vi "Save_Time_Traces_HACKforPWLDA.vi"() -> (5 "Plug in titles":string[](array[string]), 7 "Plug in values":string[](array[string]))   [LabVIEW 2010]
uses:
  Plug in sub vis/save_time _trace.ctl
  Globals/Meas_global.vi
  Globals/Plug_in_data_global.vi
  Acquisition/PWA/PWAtasksGLOBAL.vi
  Globals/LDA_meas_global_1.vi
panel:
  in  "Time Series":enum16{"Milliseconds", "Seconds"}(ring)
  in  "Full Header Info?":bool
  in  "Data Type":T1
  in  "Output Directory":path
  in  "Put each block into separate file":bool
  in  "Leave space between blocks?":bool
  in  "Precision":i16=2
  in  "Data to save":i32[](array[ring])=[1] items=["Preston (1)", "Save Nothing"]
  in  "Separation Character":string="\t"
  # "Run this VI to update the channel names"
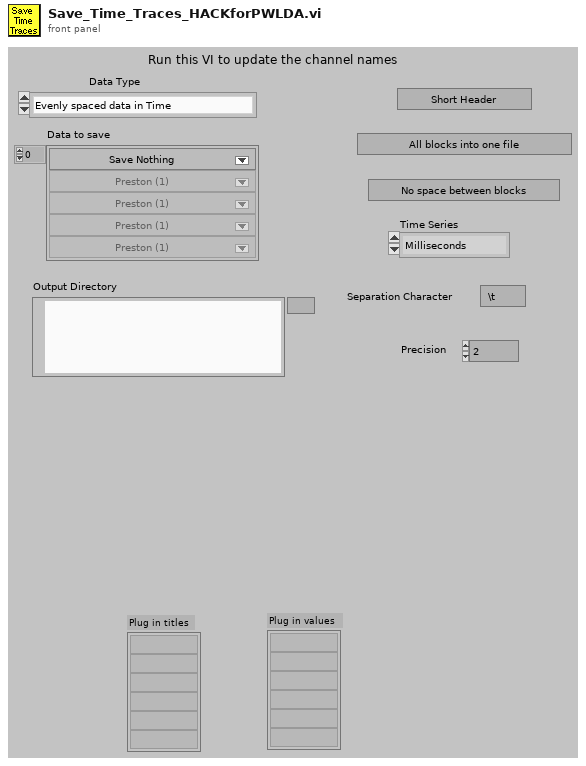
[diagram p1: front panel]
types:
  T1 = typedef "save_time _trace.ctl" = enum16{"Evenly spaced data in Time", "Unevenly spaced data in Time", "Pulsed Wire data"}
  T2 = typedef "Analysis_info_cluster.ctl" = cluster{"Colour":u32, "Inst type":T3, "Inst name":string, "Symbol":string, "Code name":string, "Extra Info":string, "Inst Array":T4, "Index":i32, "Voltage Index":i32, "Extra Titles":string[], "Extra Values":string[]}
  T3 = typedef "Inst_type.ctl" = enum16{"Propeller anemometer", "Raw voltage", "Pressure Transducer", "Pitot-static tube", "Preston tube", "Hot wire", "Cross wire 1", "Cross wire 2", "Generic Linear", "Generic Polynomial", "Generic BackPoly", "Fast FID", "Thermocouple", "Cold wire", "Pulsed Wire", "LDA Vel", "LDA Tran time", "LDA Arr time"}
  T4 = typedef "Instrument_Array.ctl" = enum16{"PWA", "LDA", "Analogue"}
  T5 = enum32{"existing file", "new file", "new or existing file", "existing dir", "new dir", "new or existing dir", "existing file (use LLBs)", "new file (use LLBs)", "new or existing file (use LLBs)", "new or existing file or directory (use LLBs)"}
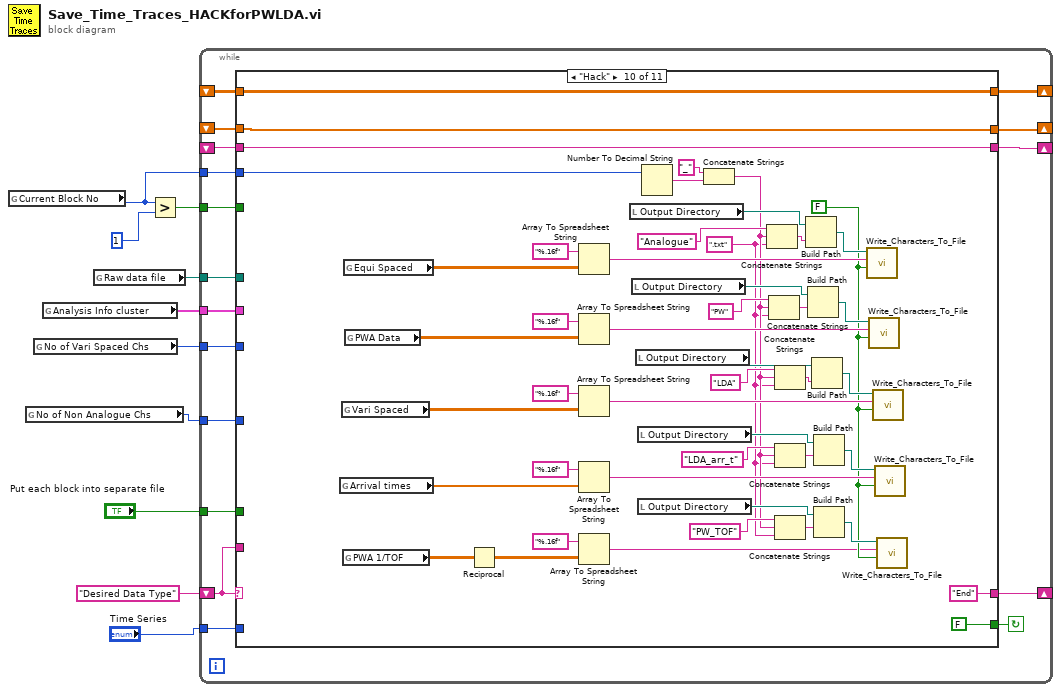
[diagram p0: block diagram]
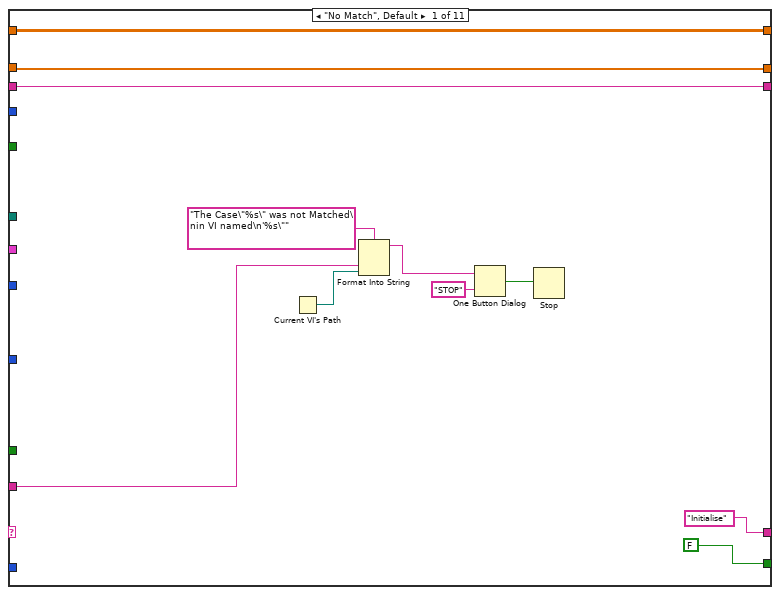
[diagram p2: hidden frame]
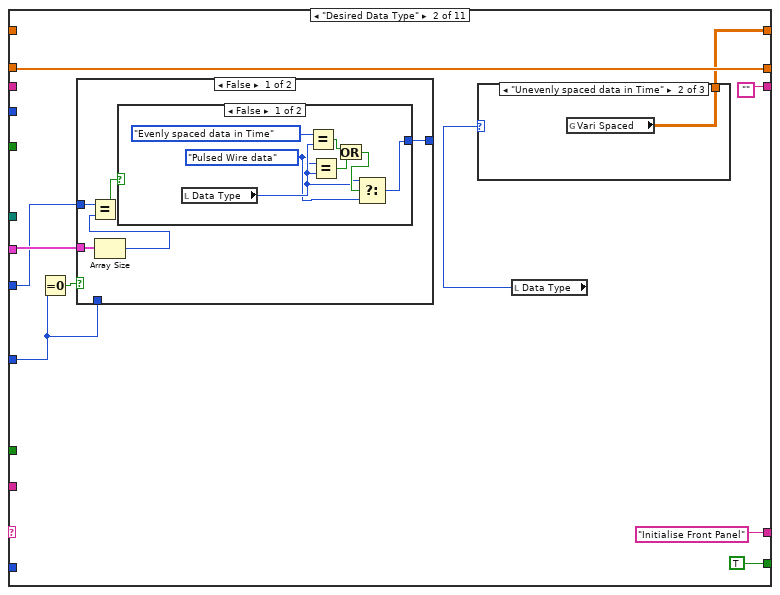
[diagram p3: hidden frame]
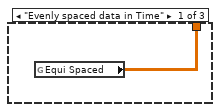
[diagram p4: hidden frame]
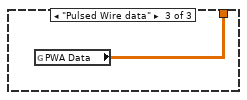
[diagram p5: hidden frame]
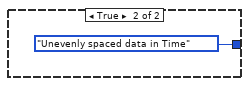
[diagram p6: hidden frame]
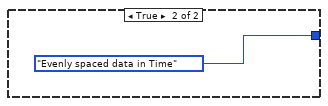
[diagram p7: hidden frame]
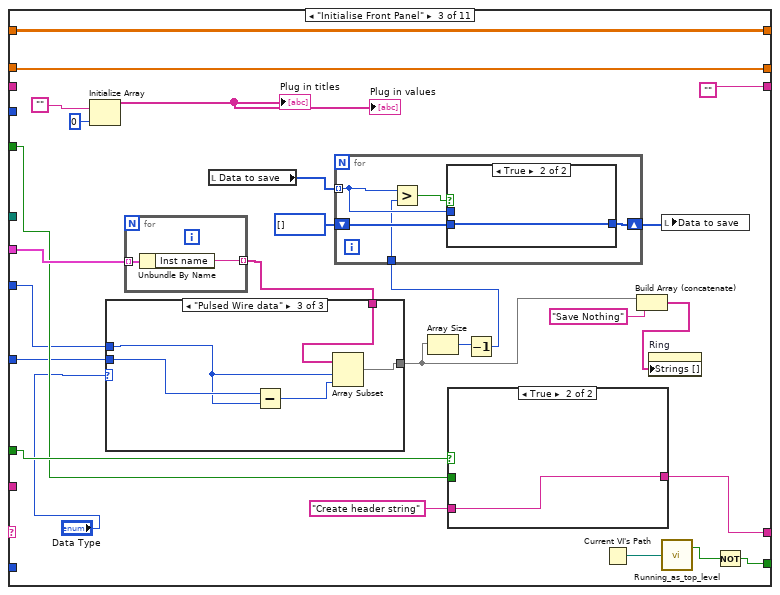
[diagram p8: hidden frame]
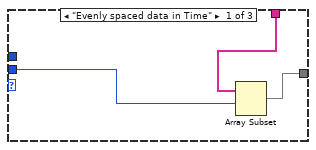
[diagram p9: hidden frame]
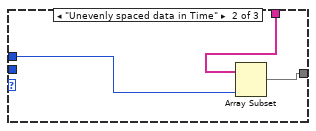
[diagram p10: hidden frame]
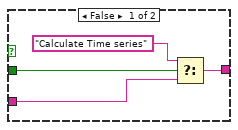
[diagram p11: hidden frame]
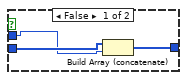
[diagram p12: hidden frame]
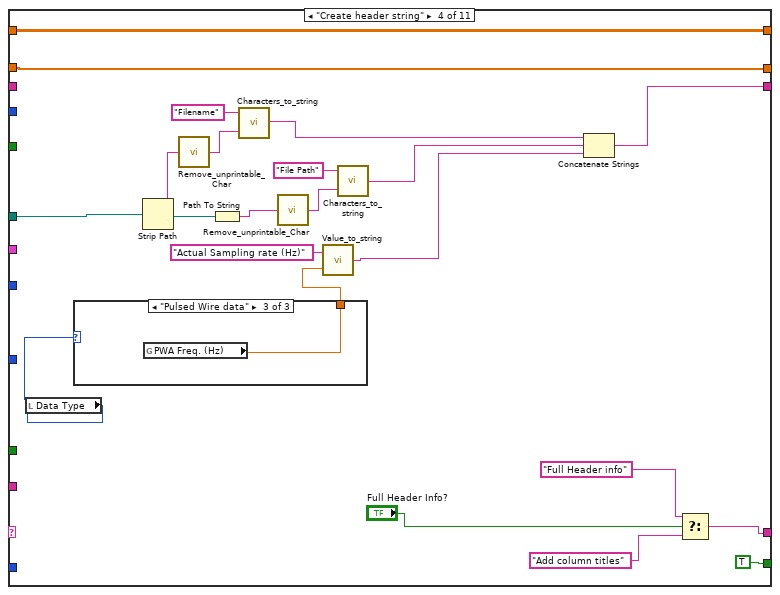
[diagram p13: hidden frame]
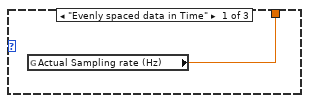
[diagram p14: hidden frame]
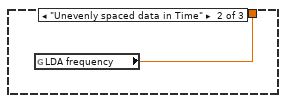
[diagram p15: hidden frame]
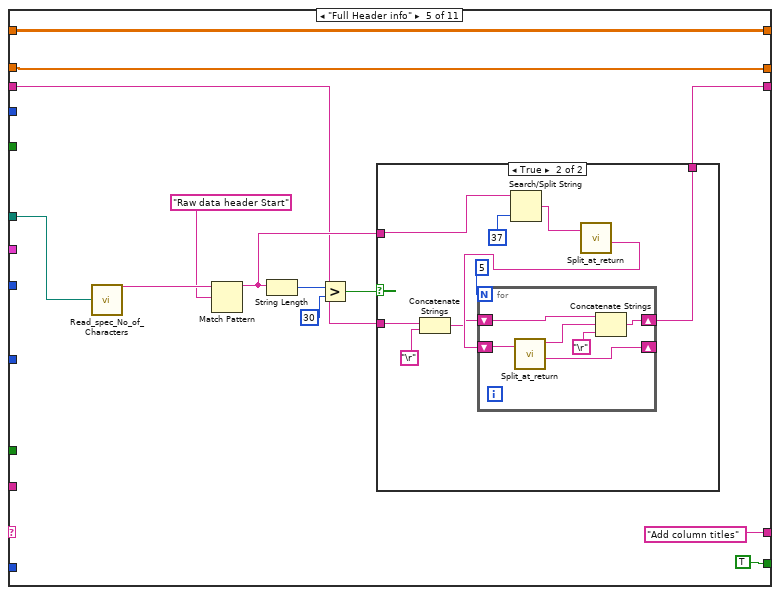
[diagram p16: hidden frame]
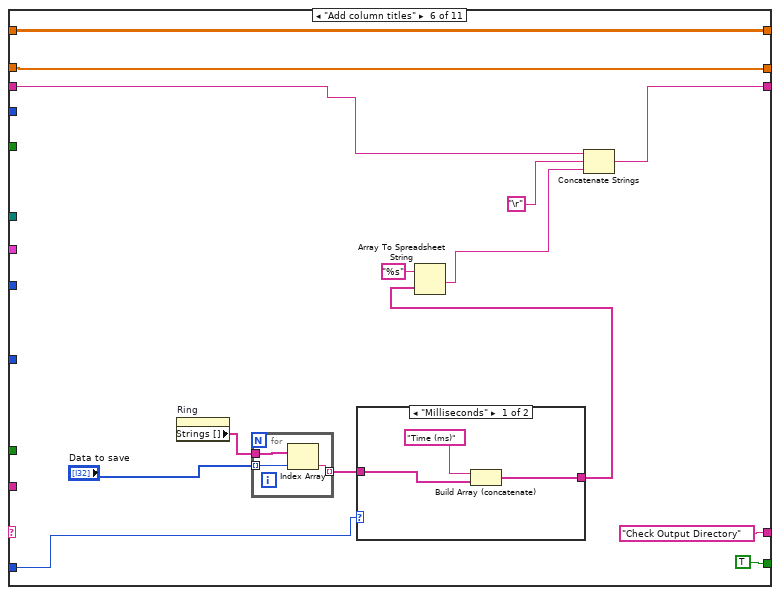
[diagram p18: hidden frame]
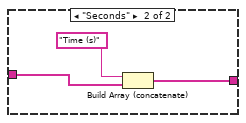
[diagram p19: hidden frame]
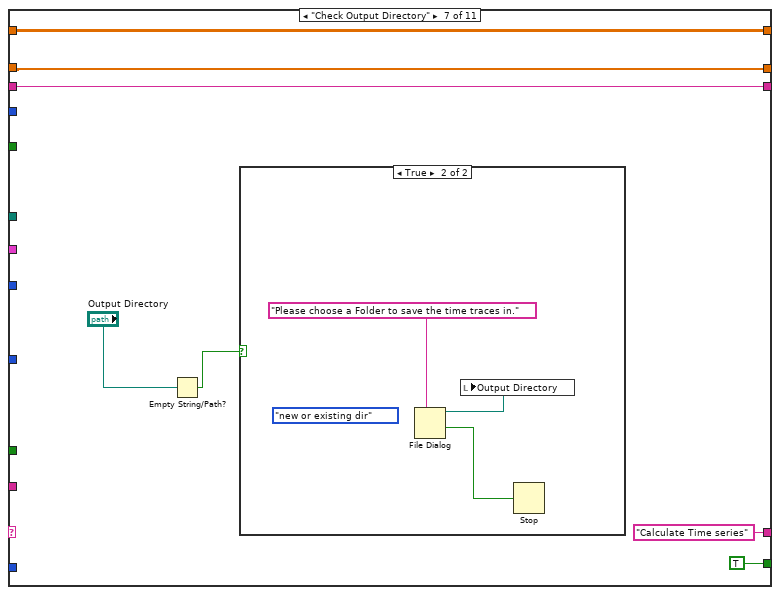
[diagram p20: hidden frame]
diagram:
  n1 = global read "Meas_global.vi" "Current Block No"() -> (w5:i32)
  n2 = global read "Meas_global.vi" "No of Non Analogue Chs"() -> (w1:i32)
  n3 = global read "Meas_global.vi" "No of Vari Spaced Chs"() -> (w3:i32)
  n4 = global read "Meas_global.vi" "Analysis Info cluster"() -> (w4:T2[])
  n5 = global read "Meas_global.vi" "Raw data file"() -> (w8:path)
  n6 = Greater?(x=w5, y=1) -> (0:w6:bool)
  n7 = while {
    shift-left: "Desired Data Type" -> [w25]
    shift-right: [w26] -> _
    shift-right: [w22] -> _
    shift-left: _ -> [w21]
    tunnel: "Put each block into separate file" -> [w24]
    tunnel: w8 -> [w23]
    tunnel: w6 -> [w20]
    shift-right: [w19] -> _
    shift-left: _ -> [w18]
    tunnel: w5 -> [w17]
    tunnel: w4 -> [w16]
    tunnel: w3 -> [w15]
    shift-right: [w14] -> _
    shift-left: _ -> [w13]
    tunnel: "Time Series" -> [w12]
    tunnel: w1 -> [w11]
    stop <- w27 continue-if-true
    n8 = case shown="\"Hack\"" w25 {
      tunnel: [FALSE TRUE w82 TRUE TRUE TRUE TRUE TRUE TRUE FALSE FALSE] -> w27
      tunnel: ["Initialise" "Initialise Front Panel" w80 w119 "Add column titles" ("t") "Check Output Directory" ("t") "Calculate Time series" ("t") "Create Columns" ("t") "Hack" ("t") "End" "End" ("t")] -> w26
      tunnel: w25 -> [w33 _ _ _ _ _ _ _ _ _ _]
      tunnel: w24 -> [_ _ w79 _ _ _ _ _ _ _ w364]
      tunnel: w23 -> [_ _ _ w130 w147 _ _ _ _ _ w380]
      tunnel: [w30 "" "" w129 w146 w183 w200 w210 w261 w334 w376] -> w22
      tunnel: w21 -> [w30 _ _ _ w145 w175 w200 w210 w263 w334 w376]
      tunnel: w20 -> [_ _ w78 _ _ _ _ _ _ _ w357]
      tunnel: [w29 w47 w90 w128 w155 w181 w197 w212 w259 w354 w367] -> w19
      tunnel: w18 -> [w29 w47 w90 w128 w155 w181 w197 _ w259 w354 w367]
      tunnel: w17 -> [_ _ _ _ _ _ _ _ _ w328 w366]
      tunnel: w16 -> [_ w44 w86 _ _ _ _ _ _ _ _]
      tunnel: w15 -> [_ w41 w68 _ _ _ _ _ _ _ _]
      tunnel: [w28 w43 w67 w125 w154 w176 w196 w208 w257 w353 w360] -> w14
      tunnel: w13 -> [w28 _ w67 w125 w154 w176 w196 w208 w257 w353 w360]
      tunnel: w12 -> [_ _ _ _ _ w173 _ w207 w256 _ _]
      tunnel: w11 -> [_ w42 w66 _ _ _ _ _ _ _ _]
      frame "No Match", Default {
        n9 = Current VI's Path() -> (path=w32:path)
        n10 = Format Into String(format string="The Case\"%s\" was not Matched\nin VI named\n'%s\"" ("Format String"), w33, w32) -> (resulting string=w36:string)  [unwired: 2 in, 1 out]
        n11 = One Button Dialog(message=w36, button name ("OK")="STOP") -> (true=w34:bool)
        n12 = Stop(stop? (T)=w34) -> ()
      }
      frame "Desired Data Type" {
        n13 = Equal To 0?(x=w42) -> (x = 0?=w46:bool)
        n14 = case shown="False" w46 {
          tunnel: [w55 save_time__trace."Evenly spaced data in Time" ("Data Type")] -> _
          tunnel: w44 -> [w56 _]
          tunnel: w42 -> [_ _]
          tunnel: w41 -> [w53 _]
          frame False {
            n15 = Array Size(array=w56) -> (size(s)=w54:i32)
            n16 = Equal?(x=w53, y=w54) -> (x = y?=w52:bool)
            n17 = case shown="False" w52 {
              tunnel: [w57 save_time__trace."Unevenly spaced data in Time" ("Data Type")] -> w55
              frame False {
                w58 = save_time__trace."Pulsed Wire data" ("Data Type")
                n18 = local read "Data Type"() -> (w59:T1)
                n19 = Equal?(x=save_time__trace."Evenly spaced data in Time" ("Data Type"), y=w59) -> (x = y?=w61:bool)
                n20 = Equal?(x=w58, y=w59) -> (x = y?=w62:bool)
                n21 = Or(x=w61, y=w62) -> (x .or. y?=w60:bool)
                n22 = Select(t=w59, s=w60, f=w58) -> (s? t:f=w57:T1)
              }
              frame True {
              }
            }
          }
          frame True {
          }
        }
        n23 = local read "Data Type"() -> (w40:T1)
        n24 = case shown="\"Unevenly spaced data in Time\"" w40 {
          tunnel: [w49 w50 w51] -> w43
          frame "Evenly spaced data in Time" {
            n25 = global read "Plug_in_data_global.vi" "Equi Spaced"() -> (w49:dbl[][])
          }
          frame "Unevenly spaced data in Time" {
            n26 = global read "Plug_in_data_global.vi" "Vari Spaced"() -> (w50:dbl[][])
          }
          frame "Pulsed Wire data" {
            n27 = global read "PWAtasksGLOBAL.vi" "PWA Data"() -> (w51:dbl[][])
          }
        }
      }
      frame "Initialise Front Panel" {
        n28 = Initialize Array("", 0) -> (→"Plug in values" →"Plug in titles":string[])
        n29 = for {
          tunnel: w86 -> [w118] mode=indexing
          tunnel: [w117] -> w72 mode=indexing
          n30 = Unbundle By Name(w118) -> ("Inst name"=w117:string)
        }
        n31 = case shown="\"Pulsed Wire data\"" "Data Type" {
          tunnel: w72 -> [w94 w97 w102]
          tunnel: [w93 w96 w101] -> w71
          tunnel: w68 -> [_ w95 w99]
          tunnel: w66 -> [w92 _ w100]
          frame "Evenly spaced data in Time" {
            n32 = Array Subset(array=w94, index=w92) -> (w93:string[])  [unwired: 1 in]
          }
          frame "Unevenly spaced data in Time" {
            n33 = Array Subset(array=w97, length=w95) -> (w96:string[])  [unwired: 1 in]
          }
          frame "Pulsed Wire data" {
            n34 = Subtract(x=w100, y=w99) -> (x-y=w98:i32)
            n35 = Array Subset(array=w102, index=w99, length=w98) -> (w101:string[])
          }
        }
        n36 = local read "Data to save"() -> (w85:i32[])
        n37 = Array Size(array=w71) -> (size(s)=w70:i32)
        n38 = case shown="True" w79 {
          tunnel: [w106 w107] -> w80
          tunnel: w78 -> [w105 _]
          tunnel: "Create header string" -> [w103 w107]
          frame False {
            n39 = Select(t="Calculate Time series", s=w105, f=w103) -> (s? t:f=w106:string)
          }
          frame True {
          }
        }
        n40 = Decrement(x=w70) -> (x-1=w69:i32)
        n41 = for {
          tunnel: w85 -> [w109] mode=indexing
          shift-right: [w110] -> w83
          shift-left: i32[] [] -> [w111]
          tunnel: w69 -> [w108]
          n42 = Greater?(x=w109, y=w108) -> (0:w112:bool)
          n43 = case shown="True" w112 {
            tunnel: w111 -> [w115 w116]
            tunnel: [w114 w116] -> w110
            tunnel: w109 -> [w113 _]
            frame False {
              n44 = Build Array (concatenate)(w115, w113) -> (w114:i32[])
            }
            frame True {
            }
          }
        }
        n45 = Current VI's Path() -> (path=w77:path)
        n46 = Build Array (concatenate)(w71, "Save Nothing") -> (w74:string[])
        n47 = property on="Ring" class="Ring (strict)"("Strings []"=w74) -> ()  [unwired: 2 in, 2 out]
        n48 = local write "Data to save"(w83) -> ()
        n49 = call "Running_as_top_level.vi"("Vi path name"=w77) -> ("Top Level"=w76:bool)  [unwired: 1 out]
        n50 = Not(x=w76) -> (.not. x?=w82:bool)
      }
      frame "Create header string" {
        n51 = local read "Data Type"() -> (w124:T1)
        n52 = case shown="\"Pulsed Wire data\"" w124 {
          tunnel: [w141 w142 w143] -> w123
          frame "Evenly spaced data in Time" {
            n53 = global read "Meas_global.vi" "Actual Sampling rate (Hz)"() -> (w141:dbl)
          }
          frame "Unevenly spaced data in Time" {
            n54 = global read "Meas_global.vi" "LDA frequency"() -> (w142:dbl)
          }
          frame "Pulsed Wire data" {
            n55 = global read "PWAtasksGLOBAL.vi" "PWA Freq. (Hz)"() -> (w143:dbl)
          }
        }
        n56 = Strip Path(path=w130) -> (stripped path=w136:path, name=w132:string)
        n57 = call "Remove_unprintable_Char.vi"("Input String"=w132) -> ("Output String"=w133:string)
        n58 = Path To String(path=w136) -> (string=w137:string)
        n59 = call "Characters_to_string.vi"("Characters to write"=w133, "Label for characters"="Filename") -> ("Output string"=w138:string)
        n60 = call "Remove_unprintable_Char.vi"("Input String"=w137) -> ("Output String"=w134:string)
        n61 = call "Value_to_string.vi"("Value"=w123, "Label for value"="Actual Sampling rate (Hz)") -> ("Output string"=w126:string)  [unwired: 1 in]
        n62 = call "Characters_to_string.vi"("Characters to write"=w134, "Label for characters"="File Path") -> ("Output string"=w139:string)
        n63 = Concatenate Strings(w138, w139, w126) -> (w129:string)
        n64 = Select(t="Full Header info", s="Full Header Info?", f="Add column titles" ("t")) -> (s? t:f=w119:string)
      }
      frame "Full Header info" {
        n65 = call "Read_spec_No_of_Characters.vi"("Filename"=w147) -> ("character string"=w153:string)  [unwired: 1 out]
        n66 = Match Pattern(string=w153, regular expression="Raw data header Start") -> (before substring=w149:string)  [unwired: 4 out]
        n67 = String Length(string=w149) -> (length=w148:i32)
        n68 = Greater?(x=w148, y=30) -> (0:w150:bool)
        n69 = case shown="True" w150 {
          tunnel: w149 -> [_ w165]
          tunnel: w145 -> [w157 w160]
          tunnel: [w157 w163] -> w146
          frame False {
          }
          frame True {
            n70 = Concatenate Strings(w160, "\r") -> (w159:string)
            n71 = Search/Split String(string=w165, offset (0)=37 ("y")) -> (match + rest of string=w162:string)  [unwired: 3 out]
            n72 = call "Split_at_return.vi"("String"=w162) -> ("after substring"=w161:string)  [unwired: 1 in, 3 out]
            n73 = for {
              N: 5 -> [_]
              shift-right: [w170] -> w163
              shift-left: w159 -> [w172]
              shift-right: [w168] -> _
              shift-left: w161 -> [w169]
              n74 = call "Split_at_return.vi"("String"=w169) -> ("before substring"=w171:string, "after substring"=w168:string)  [unwired: 1 in, 2 out]
              n75 = Concatenate Strings(w172, w171, "\r") -> (w170:string)
            }
          }
        }
      }
      frame "Add column titles" {
        n76 = property on="Ring" class="Ring (strict)"() -> ("Strings []"=w178:string[])  [unwired: 2 in, 2 out]
        n77 = for {
          tunnel: w178 -> [w189]
          tunnel: "Data to save" -> [w188] mode=indexing
          tunnel: [w187] -> w177 mode=indexing
          n78 = Index Array(array=w189, index=w188) -> (element=w187:string)
        }
        n79 = case shown="\"Milliseconds\"" w173 {
          tunnel: w177 -> [w192 w195]
          tunnel: [w191 w194] -> w185
          frame "Milliseconds" {
            n80 = Build Array (concatenate)("Time (ms)", w192) -> (w191:string[])
          }
          frame "Seconds" {
            n81 = Build Array (concatenate)("Time (s)", w195) -> (w194:string[])
          }
        }
        n82 = Array To Spreadsheet String(array=w185, 3:"%s" ("format string")) -> (spreadsheet string=w179:string)  [unwired: 1 out]
        n83 = Concatenate Strings(w175, "\r", w179) -> (w183:string)
      }
      frame "Check Output Directory" {
        n84 = Empty String/Path?(string/path="Output Directory") -> (empty?=w201:bool)
        n85 = case shown="True" w201 {
          frame False {
          }
          frame True {
            (unwired) T5."new or existing dir" ("select mode (2)")
            n86 = File Dialog(7:"Please choose a Folder to save the time traces in." ("prompt")) -> (1:w204:bool, 3:w205:path)  [unwired: 1 in, 7 out]
            n87 = local write "Output Directory"(w205) -> ()
            n88 = Stop(stop? (T)=w204) -> ()
          }
        }
      }
      frame "Calculate Time series" {
        n89 = local read "Data Type"() -> (w209:T1)
        n90 = case shown="\"Milliseconds\"" w207 {
          tunnel: [1.0 0.001] -> w206
          frame "Milliseconds" {
          }
          frame "Seconds" {
          }
        }
        n91 = case shown="\"Pulsed Wire data\"" w209 {
          tunnel: [w222 w237 w247] -> w212
          tunnel: w208 -> [w220 w235 _]
          tunnel: w206 -> [w216 w232 w246]
          frame "Evenly spaced data in Time" {
            n92 = global read "Meas_global.vi" "Actual Sampling rate (Hz)"() -> (w217:dbl)
            n93 = Reciprocal(x=w217) -> (1/x=w225:dbl)
            n94 = Array Size(array=w220) -> (size(s)=w221:i32[])
            n95 = Multiply(x=w225, y=1000.0) -> (x*y=w223:dbl)
            n96 = Index Array(array=w221, index=1) -> (element=w218:i32)
            n97 = for {
              N: w218 -> [_]
              tunnel: w223 -> [w229]
              tunnel: [w227] -> w222 mode=indexing
              tunnel: w216 -> [w226]
              i -> [w230]
              n98 = Multiply(x=w229, y=w230) -> (x*y=w228:dbl)
              n99 = Multiply(x=w228, y=w226) -> (x*y=w227:dbl)
            }
          }
          frame "Pulsed Wire data" {
            n100 = global read "PWAtasksGLOBAL.vi" "PWA Freq. (Hz)"() -> (w231:dbl)
            n101 = Reciprocal(x=w231) -> (1/x=w240:dbl)
            n102 = Array Size(array=w235) -> (size(s)=w236:i32[])
            n103 = Multiply(x=w240, y=1000.0) -> (x*y=w238:dbl)
            n104 = Index Array(array=w236, index=1) -> (element=w233:i32)
            n105 = for {
              N: w233 -> [_]
              tunnel: w238 -> [w244]
              tunnel: [w242] -> w237 mode=indexing
              tunnel: w232 -> [w241]
              i -> [w245]
              n106 = Multiply(x=w244, y=w245) -> (x*y=w243:dbl)
              n107 = Multiply(x=w243, y=w241) -> (x*y=w242:dbl)
            }
          }
          frame "Unevenly spaced data in Time" {
            n108 = global read "LDA_meas_global_1.vi" "Arrival times"() -> (w249:dbl[])
            n109 = for {
              shift-right: [w252] -> _
              shift-left: 0.0 -> [w254]
              tunnel: w249 -> [w253] mode=indexing
              tunnel: [w251] -> w247 mode=indexing
              tunnel: w246 -> [w250]
              n110 = Add(x=w254, y=w253) -> (x+y=w252:dbl)
              n111 = Multiply(x=w252, y=w250) -> (x*y=w251:dbl)
            }
          }
        }
      }
      frame "Create Columns" {
        (unwired) "Write File"
        n112 = local read "Data to save"() -> (w258:i32[])
        n113 = Array Size(array=w258) -> (size(s)=w266:i32)
        n114 = Decrement(x=w266) -> (x-1=w267:i32)
        n115 = for {
          shift-right: [w280] -> w262
          shift-left: "" -> [w274]
          tunnel: "Separation Character" -> [w270]
          tunnel: w258 -> [w278]
          tunnel: w257 -> [w277]
          tunnel: w267 -> [w273]
          tunnel: w259 -> [w269] mode=indexing
          tunnel: w256 -> [w268]
          i -> [w271]
          n116 = Index Array(array=w277, index (col)=w271) -> (element=w276:dbl[])  [unwired: 1 in]
          n117 = case shown="\"Seconds\"" w268 {
            tunnel: [w285 w289] -> w281
            tunnel: w270 -> [w284 w288]
            tunnel: w269 -> [w283 w287]
            frame "Seconds" {
              n118 = Format Into String(format string="%.4f%s", w283, w284) -> (resulting string=w285:string)  [unwired: 2 in, 1 out]
            }
            frame "Milliseconds" {
              n119 = Format Into String(format string="%.1f%s", w287, w288) -> (resulting string=w289:string)  [unwired: 2 in, 1 out]
            }
          }
          n120 = for {
            shift-right: [w298] -> w275
            shift-left: w281 -> [w300]
            tunnel: w270 -> [w297]
            tunnel: w278 -> [w296] mode=indexing
            tunnel: w276 -> [w295]
            tunnel: w273 -> [w292]
            tunnel: "Precision" -> [w290]
            i -> [w293]
            n121 = Index Array(array=w295, index=w296) -> (element=w294:dbl)
            n122 = Equal?(x=w293, y=w292) -> (x = y?=w291:bool)
            n123 = Number To Fractional String(number=w294, precision (6)=w290) -> (F-format string=w299:string)  [unwired: 2 out]
            n124 = case shown="True" w291 {
              tunnel: w300 -> [w304 w307]
              tunnel: w299 -> [w303 w306]
              tunnel: [w302 w305] -> w298
              tunnel: w297 -> [w301 _]
              frame False {
                n125 = Concatenate Strings(w304, w303, w301) -> (w302:string)
              }
              frame True {
                n126 = Concatenate Strings(w307, w306) -> (w305:string)
              }
            }
          }
          n127 = Concatenate Strings(w274, w275, "\r") -> (w280:string)
        }
        n128 = Concatenate Strings(w263, w262) -> (w261:string)
      }
      frame "Hack" {
        w312 = ".txt" ("string")
        w311 = FALSE ("append to file? (new file:F)")
        n129 = global read "LDA_meas_global_1.vi" "Arrival times"() -> (w333:dbl[])
        n130 = global read "Plug_in_data_global.vi" "Vari Spaced"() -> (w332:dbl[][])
        n131 = global read "PWAtasksGLOBAL.vi" "PWA 1/TOF"() -> (w308:dbl[][])
        n132 = global read "Plug_in_data_global.vi" "Equi Spaced"() -> (w330:dbl[][])
        n133 = global read "PWAtasksGLOBAL.vi" "PWA Data"() -> (w331:dbl[][])
        n134 = Reciprocal(x=w308) -> (1/x=w309:dbl[][])
        n135 = Array To Spreadsheet String(array=w330, 3:"%.16f" ("format string")) -> (spreadsheet string=w346:string)  [unwired: 1 out]
        n136 = Array To Spreadsheet String(array=w331, 3:"%.16f" ("format string")) -> (spreadsheet string=w336:string)  [unwired: 1 out]
        n137 = Array To Spreadsheet String(array=w332, 3:"%.16f" ("format string")) -> (spreadsheet string=w338:string)  [unwired: 1 out]
        n138 = Array To Spreadsheet String(array=w333, 3:"%.16f" ("format string")) -> (spreadsheet string=w337:string)  [unwired: 1 in]
        n139 = Array To Spreadsheet String(array=w309, 3:"%.16f" ("format string")) -> (spreadsheet string=w310:string)  [unwired: 1 out]
        n140 = local read "Output Directory"() -> (w345:path)
        n141 = local read "Output Directory"() -> (w343:path)
        n142 = local read "Output Directory"() -> (w342:path)
        n143 = local read "Output Directory"() -> (w339:path)
        n144 = local read "Output Directory"() -> (w315:path)
        n145 = Number To Decimal String(number=w328) -> (decimal integer string=w327:string)  [unwired: 1 out]
        n146 = Concatenate Strings("_" ("string"), w327) -> (w313:string)
        n147 = Concatenate Strings("Analogue" ("string"), w313, w312) -> (w329:string)
        n148 = Concatenate Strings("PW" ("string"), w313, w312) -> (w324:string)
        n149 = Concatenate Strings("LDA" ("string"), w313, w312) -> (w323:string)
        n150 = Concatenate Strings("LDA_arr_t" ("string"), w313, w312) -> (w325:string)
        n151 = Concatenate Strings("PW_TOF" ("string"), w313, w312) -> (w316:string)
        n152 = Build Path(base path=w345, name or relative path=w329) -> (appended path=w344:path)
        n153 = Build Path(base path=w343, name or relative path=w324) -> (appended path=w335:path)
        n154 = Build Path(base path=w342, name or relative path=w323) -> (appended path=w341:path)
        n155 = Build Path(base path=w339, name or relative path=w325) -> (appended path=w340:path)
        n156 = Build Path(base path=w315, name or relative path=w316) -> (appended path=w314:path)
        n157 = call "Write_Characters_To_File.vi"("file path (dialog if empty)"=w344, "character string"=w346, "append to file? (new file:F)"=w311) -> ()  [unwired: 2 in, 4 out]
        n158 = call "Write_Characters_To_File.vi"("file path (dialog if empty)"=w335, "character string"=w336, "append to file? (new file:F)"=w311) -> ()  [unwired: 2 in, 4 out]
        n159 = call "Write_Characters_To_File.vi"("file path (dialog if empty)"=w341, "character string"=w338, "append to file? (new file:F)"=w311) -> ()  [unwired: 2 in, 4 out]
        n160 = call "Write_Characters_To_File.vi"("file path (dialog if empty)"=w340, "character string"=w337, "append to file? (new file:F)"=w311) -> ()  [unwired: 2 in, 4 out]
        n161 = call "Write_Characters_To_File.vi"("file path (dialog if empty)"=w314, "character string"=w310, "append to file? (new file:F)"=w311) -> ()  [unwired: 2 in, 4 out]
      }
      frame "Write File" {
        n162 = Strip Path(path=w380) -> (stripped path=w361:path, name=w355:string)
        n163 = call "Add_filename_suffix.vi"("Filename"=w355) -> ("Base name"=w356:string)  [unwired: 1 in, 3 out]
        n164 = case shown="True" w364 {
          tunnel: w356 -> [w387 w390]
          tunnel: w366 -> [_ w395]
          tunnel: [w386 w393] -> w365
          tunnel: w357 -> [w384 _]
          tunnel: [w384 FALSE] -> w363
          tunnel: [w383 w389] -> w362
          tunnel: w361 -> [w383 w391]
          tunnel: [2 ("y") 3 ("y")] -> w359
          frame False {
            n165 = Concatenate Strings(w387, ".xls" ("string")) -> (w386:string)
          }
          frame True {
            n166 = Format Into String(format string="_%d.xls", initial string=w390, w395) -> (resulting string=w393:string)  [unwired: 1 in, 1 out]
            n167 = Build Path(base path=w391, name or relative path=w390) -> (appended path=w389:path)
          }
        }
        n168 = Build Path(base path=w362, name or relative path=w365) -> (appended path=w381:path)
        n169 = Path to Array of Strings(0:w381) -> (2:w373:string[])  [unwired: 1 out]
        n170 = Array Size(array=w373) -> (size(s)=w372:i32)
        n171 = local read "Output Directory"() -> (w369:path)
        n172 = Subtract(x=w372, y=w359) -> (x-y=w371:i32)
        n173 = Not(x=w357) -> (.not. x?=w358:bool)
        n174 = Array Subset(array=w373, index=w371) -> (w370:string[])  [unwired: 1 in]
        n175 = call "Build_Pathname.vi"("Output Array"=w370, "Pathname"=w369) -> ("Appended path"=w368:path)
        n176 = case shown="True" w363 {
          tunnel: [w396 w404] -> w378
          tunnel: w376 -> [w396 w403]
          tunnel: [w399 w402] -> w379
          tunnel: w368 -> [w398 w400]
          tunnel: [w397 w400] -> w377
          frame False {
            w399 = FALSE  # append to file? (new file:F)
            n177 = call "Create_directory_path.vi"("Path name"=w398) -> ("Path name Out"=w397:path)
          }
          frame True {
            w402 = TRUE  # append to file? (new file:F)
            n178 = case shown="True" "Leave space between blocks?" {
              tunnel: [w405 w408] -> w404
              tunnel: w403 -> [w405 w407]
              frame False {
              }
              frame True {
                n179 = Concatenate Strings("\r", w407) -> (w408:string)
              }
            }
          }
        }
        n180 = call "Write_Characters_To_File.vi"("file path (dialog if empty)"=w377, "advisory dialog? (display:T)"=w358, "character string"=w378, "append to file? (new file:F)"=w379) -> ()  [unwired: 1 in, 4 out]
      }
    }
  }
